vi "_set_parameters_CAUTION.vi"(8 "error in (no error)":errorcluster, 10 "a_pDeviceParm":u8[](array[numeric]), 11 "UV-VIS_AVANTES in":refnum<class "UV-VIS_AVANTES.lvclass">) -> (0 "error out":errorcluster, 3 "UV-VIS_AVANTES out":refnum<class "UV-VIS_AVANTES.lvclass">)   [LabVIEW 2020, in "UV-VIS_AVANTES.lvclass"]
uses:
  UV-VIS_AVANTES.lvclass
  C:/dev/TRANCON/Classes/Detector/Detector.lvclass
  Detector.lvclass/Detector.ctl
  UV-VIS_AVANTES.lvclass/UV-VIS_AVANTES.ctl
  Detector.lvclass
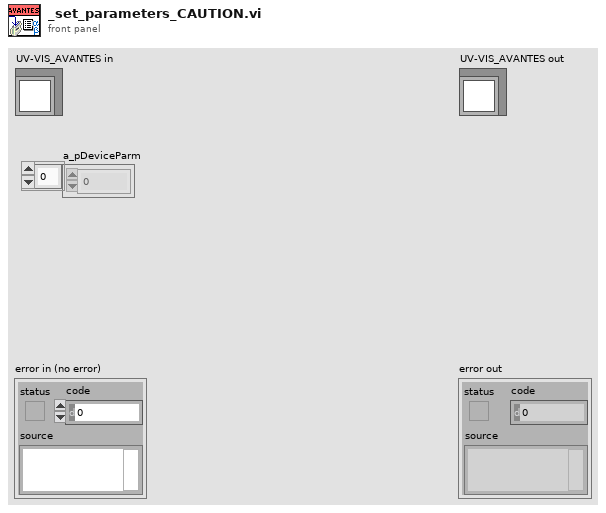
[diagram p1: front panel]
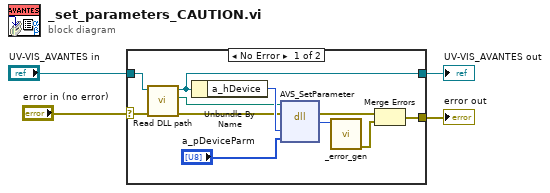
[diagram p0: block diagram]
diagram:
  n1 = case shown="No Error" "error in (no error)" {
    selector: "error in (no error)" -> [w14 w17]
    tunnel: [w5 w17] -> w3
    tunnel: [w13 w16] -> w1
    tunnel: "UV-VIS_AVANTES in" -> [w15 w16]
    frame No Error {
      n2 = call "Read DLL path.vi"("error in (no error)"=w14, "Detector in"=w15) -> ("error out"=w10:errorcluster, "DLL path"=w9:path, "Detector out"=w13:refnum<class "UV-VIS_AVANTES.lvclass">)  [unwired: 7 in]
      n3 = Unbundle By Name(w13) -> ("a_hDevice"=w11:i32)
      n4 = dll-call lib="C:/AvaSpecX64-DLL_9.4/examples/LabView/LabViewSingleChan/avaspec.dll" fn="AVS_SetParameter"(path in=w9, error in=w10, "a_hDevice"=w11, "a_pDeviceParm"="a_pDeviceParm") -> (error out=w6:errorcluster, "return type"=w7:i32)  [unwired: 3 in, 1 out]
      n5 = call "_error_gen.vi"("return type"=w7) -> ("error out"=w8:errorcluster)  [unwired: 10 in]
      n6 = Merge Errors(w6, w8) -> (w5:errorcluster)
    }
    frame Error {
    }
  }
  "error out" <- w3
  "UV-VIS_AVANTES out" <- w1
